vi "Write BMS Data.vi"(8 "error in (no error)":errorcluster, 10 "BMS Data":T1, 11 "Orion_BMS in":refnum<class "Orion_BMS.lvclass">) -> (0 "error out":errorcluster, 3 "Orion_BMS out":refnum<class "Orion_BMS.lvclass">)   [LabVIEW 2017, in "Orion_BMS.lvclass"]
uses:
  Orion_BMS.lvclass
  TypeDef_BMSData.ctl
  TypeDef_BMS_Status.ctl
  Orion_BMS.lvclass/Orion_BMS.ctl
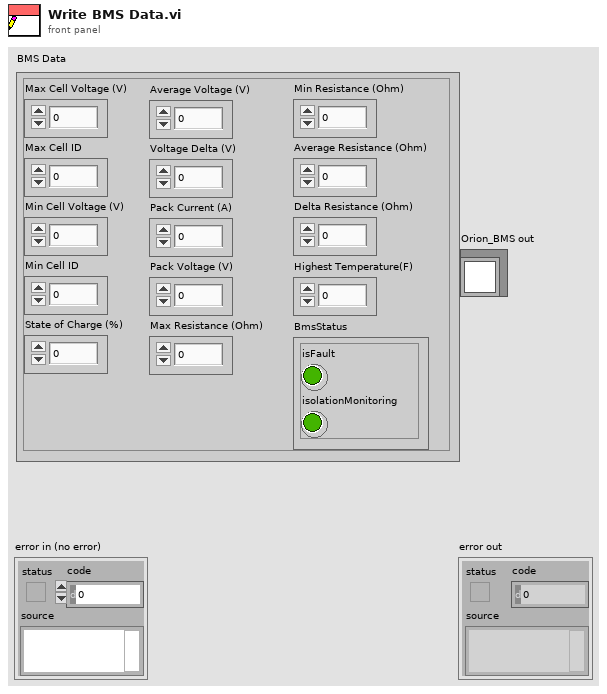
[diagram p1: front panel]
types:
  T1 = typedef "TypeDef_BMSData.ctl" = cluster{"Max Cell Voltage (V)":dbl, "Max Cell ID":dbl, "Min Cell Voltage (V)":dbl, "Min Cell ID":dbl, "State of Charge (%)":dbl, "Average Voltage (V)":dbl, "Voltage Delta (V)":dbl, "Pack Current (A)":dbl, "Pack Voltage (V)":dbl, "Max Resistance (Ohm)":dbl, "Min Resistance (Ohm)":dbl, "Average Resistance (Ohm)":dbl, "Delta Resistance (Ohm)":dbl, "Highest Temperature(F)":dbl, "BmsStatus":T2}
  T2 = typedef "TypeDef_BMS_Status.ctl" = cluster{"isFault":bool, "isolationMonitoring":bool}
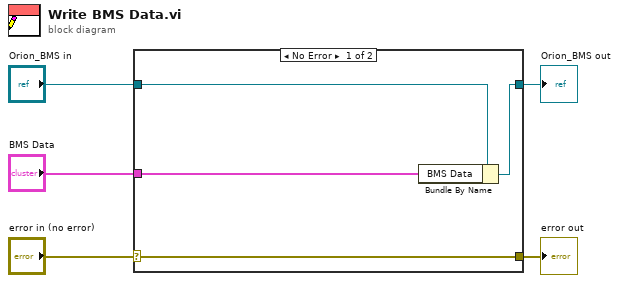
[diagram p0: block diagram]
diagram:
  n1 = case shown="No Error" "error in (no error)" {
    selector: "error in (no error)" -> [w9 w10]
    tunnel: [w9 w10] -> w4
    tunnel: [w7 w11] -> w2
    tunnel: "Orion_BMS in" -> [w8 w11]
    tunnel: "BMS Data" -> [w6 _]
    frame No Error {
      n2 = Bundle By Name(cluster=w8, "BMS Data"=w6) -> (w7:refnum<class "Orion_BMS.lvclass">)
    }
    frame Error {
    }
  }
  "error out" <- w4
  "Orion_BMS out" <- w2
